vi "SubVI-string.vi"(8 "Separator (,)":string=",", 9 "Strings In":string[](array[string])=["a", "b", "c"]) -> (0 "String":string)   [LabVIEW 2022 SP3]
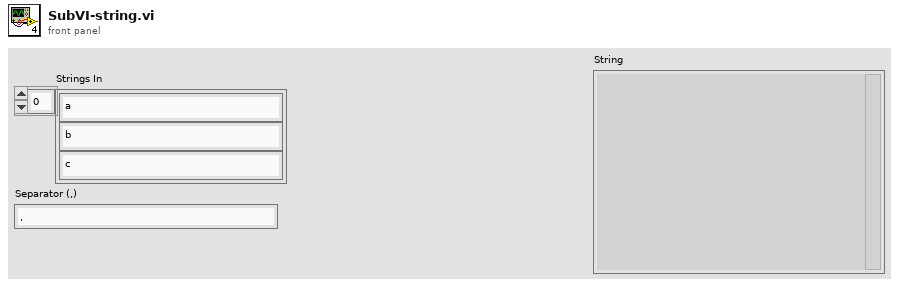
[diagram p1: front panel]
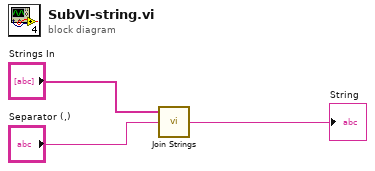
[diagram p0: block diagram]
diagram:
  n1 = call <vilib>:"Join Strings.vi"("Separator (,)"="Separator (,)", "Strings In"="Strings In") -> ("String"=→"String":string)  [unwired: 1 in]
